vi "IPI_Cal_Laser_Y_Pos.vi"(10 "Y Distance":string, 11 "Y pos":dbl[](array[numeric])) -> (3 "Y Laser Pos":dbl[](array[numeric]))   [LabVIEW 2015]
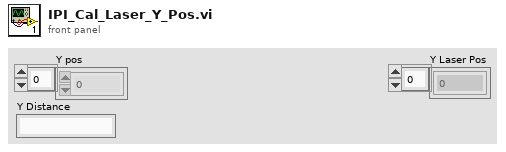
[diagram p1: front panel]
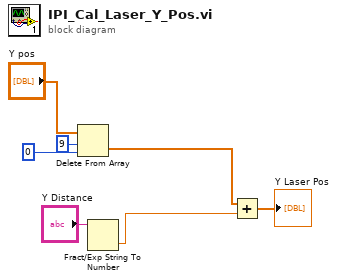
[diagram p0: block diagram]
diagram:
  n1 = Delete From Array(array="Y pos", length=9 ("长度"), index=0 ("索引")) -> (deleted portion=w3:dbl[])  [unwired: 1 out]
  n2 = Fract/Exp String To Number(string="Y Distance") -> (number=w2:dbl)  [unwired: 3 in, 1 out]
  n3 = Add(x=w3, y=w2) -> (x+y=→"Y Laser Pos":dbl[])
